vi "CMD_SETLOG.vi"(6 "Gantry Class in":refnum<class "Gantry.lvclass">, 7 "Console Log in":refnum<class "Console Log.lvclass">, 8 "error in (no error)":errorcluster, 10 "Arguments":string[](array[string]), 11 "gScript Interpreter in":refnum<class "gScript Interpreter.lvclass">) -> (0 "error out":errorcluster, 3 "gScript Interpreter out":refnum<class "gScript Interpreter.lvclass">, 4 "Gantry Class out":refnum<class "Gantry.lvclass">, 5 "Console Log out":refnum<class "Console Log.lvclass">)   [LabVIEW 2023, in "gScript Interpreter.lvclass"]
uses:
  gScript Interpreter.lvclass
  Application Utilities/Console Log/Console Log.lvclass
  Shared Components/Gantry Class/Gantry.lvclass
  Shared Components/FlexWorktable/FlexWorktable.lvclass
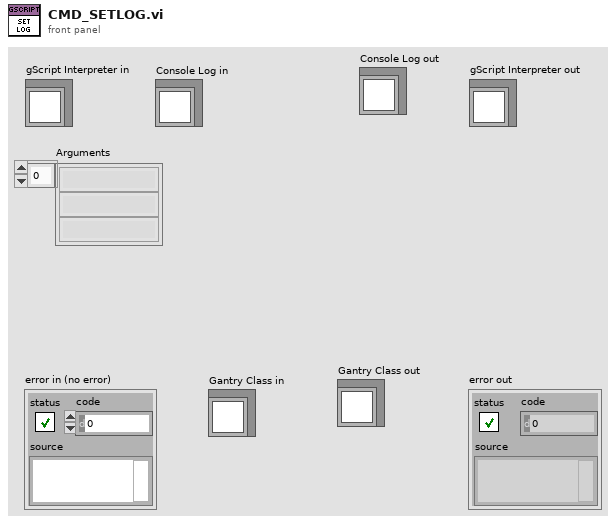
[diagram p1: front panel]
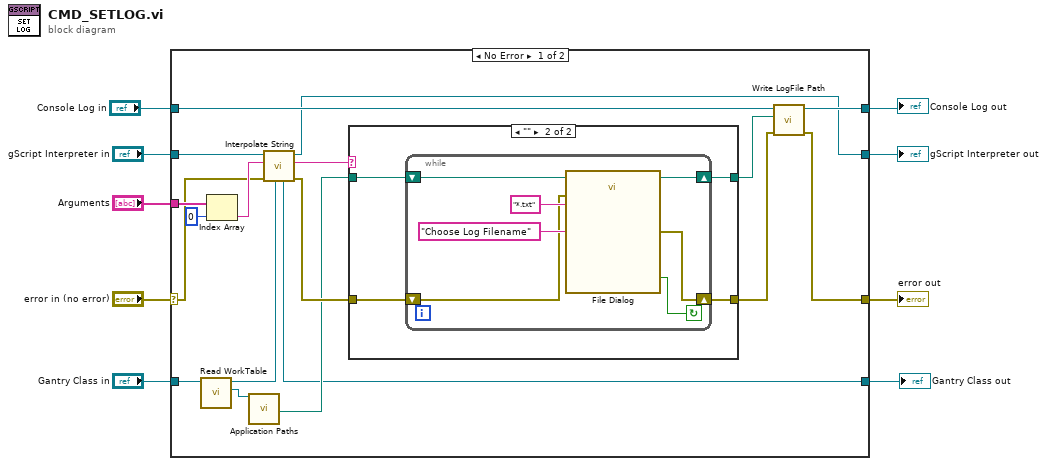
[diagram p0: block diagram]
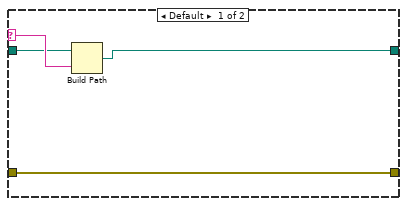
[diagram p2: hidden frame]
diagram:
  n1 = case shown="No Error" "error in (no error)" {
    selector: "error in (no error)" -> [w19 w46]
    tunnel: [w23 w46] -> w8
    tunnel: [w17 w45] -> w6
    tunnel: "gScript Interpreter in" -> [w18 w45]
    tunnel: "Arguments" -> [w27 _]
    tunnel: "Console Log in" -> [w25 w44]
    tunnel: [w24 w44] -> w3
    tunnel: "Gantry Class in" -> [w14 w43]
    tunnel: [w10 w43] -> w1
    frame No Error {
      n2 = call-dynamic "Read WorkTable.vi"("Gantry Class in"=w14) -> ("Worktable"=w13:refnum<class "FlexWorktable.lvclass">, "Gantry Class out"=w11:refnum<class "Gantry.lvclass">)  [unwired: 8 in, 1 out]
      n3 = Index Array(array=w27, index=0) -> (element=w20:string)
      n4 = call "Application Paths.vi"("FlexWorktable in"=w13) -> ("Logs Path"=w12:path)  [unwired: 12 in, 6 out]
      n5 = call-dynamic "Interpolate String.vi"("Gantry in"=w11, "error in (no error)"=w19, "Input String"=w20, "gScript Interpreter in"=w18) -> ("error out"=w15:errorcluster, "Output String"=w16:string, "gScript Interpreter out"=w17:refnum<class "gScript Interpreter.lvclass">, "Gantry out"=w10:refnum<class "Gantry.lvclass">)  [unwired: 4 in]
      n6 = case shown="\"\"" w16 {
        selector: w16 -> [w31 _]
        tunnel: w12 -> [w30 w34]
        tunnel: w15 -> [w28 w35]
        tunnel: [w28 w33] -> w21
        tunnel: [w29 w32] -> w22
        frame Default {
          n7 = Build Path(base path=w30, name or relative path=w31) -> (appended path=w29:path)
        }
        frame "" {
          n8 = while {
            shift-right: [w36] -> w33
            shift-left: w35 -> [w40]
            shift-right: [w38] -> w32
            shift-left: w34 -> [w39]
            stop <- w37 continue-if-true
            n9 = call "File Dialog"("start path"=w39, "prompt"="Choose Log Filename", "error in"=w40, "pattern (all files)"="*.txt" ("pattern label")) -> ("selected path"=w38:path, "cancelled"=w37:bool, "error out"=w36:errorcluster)  [unwired: 8 in, 1 out]
          }
        }
      }
      n10 = call-dynamic "Write LogFile Path.vi"("error in"=w21, "Log Filename"=w22, "Console Log in"=w25) -> ("error out"=w23:errorcluster, "Console Log out"=w24:refnum<class "Console Log.lvclass">)  [unwired: 7 in]
    }
    frame Error {
    }
  }
  "error out" <- w8
  "gScript Interpreter out" <- w6
  "Console Log out" <- w3
  "Gantry Class out" <- w1
